vi "Data_select.vi"(8 "m":i32=2, 9 "P":i32=64, 10 "d(k) in":dbl[][](array[numeric]), 11 "g(k) in":dbl[][](array[numeric])) -> (1 "d(k) lineal":ext[](array[numeric]), 3 "g(k) lineal":ext[](array[numeric]))   [LabVIEW 2015]
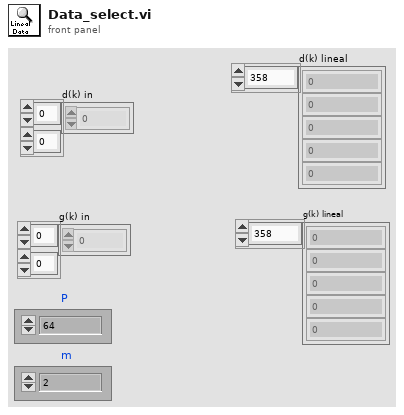
[diagram p1: front panel]
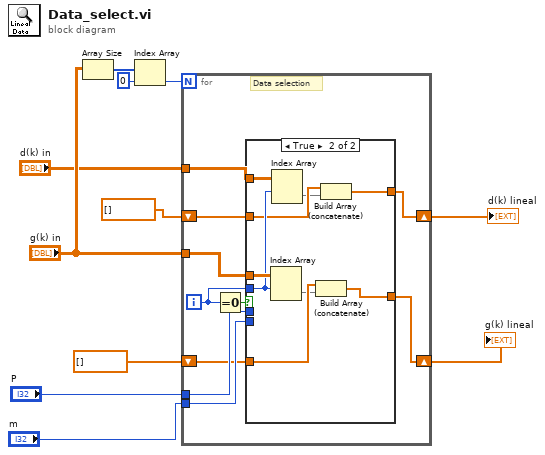
[diagram p0: block diagram]
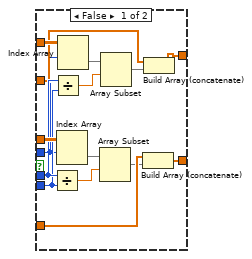
[diagram p2: hidden frame]
diagram:
  n1 = Array Size(array="g(k) in") -> (size(s)=w10:i32[])
  n2 = Index Array(array=w10, index=0) -> (element=w8:i32)
  n3 = for {
    N: w8 -> [_]
    tunnel: "g(k) in" -> [w20]
    tunnel: "m" -> [w18]
    tunnel: "P" -> [w17]
    shift-right: [w15] -> w4
    shift-left: ext[] [] ("Photon trace A") -> [w16]
    tunnel: "d(k) in" -> [w14]
    shift-right: [w12] -> w1
    shift-left: ext[] [] ("Photon trace A") -> [w13]
    i -> [w19]
    # "Data selection"
    n4 = Equal To 0?(x=w19) -> (x = 0?=w21:bool)
    n5 = case shown="True" w21 {
      tunnel: w20 -> [w36 w45]
      tunnel: w19 -> [w22 w40]
      tunnel: w18 -> [w25 _]
      tunnel: w17 -> [w26 _]
      tunnel: w16 -> [w34 w44]
      tunnel: [w35 w42] -> w15
      tunnel: w14 -> [w27 w41]
      tunnel: w13 -> [w23 w39]
      tunnel: [w24 w37] -> w12
      frame False {
        n6 = Divide(x=w26, y=w25) -> (x/y=w32:dbl)
        n7 = Divide(x=w26, y=w25) -> (x/y=w29:dbl)
        n8 = Index Array(array=w36, index (row)=w22) -> (element=w33:dbl[])  [unwired: 1 in]
        n9 = Index Array(array=w27, index (row)=w22) -> (element=w30:dbl[])  [unwired: 1 in]
        n10 = Array Subset(array=w33, index=w32) -> (w31:dbl[])  [unwired: 1 in]
        n11 = Array Subset(array=w30, index=w29) -> (w28:dbl[])  [unwired: 1 in]
        n12 = Build Array (concatenate)(w34, w31) -> (w35:ext[])
        n13 = Build Array (concatenate)(w23, w28) -> (w24:ext[])
      }
      frame True {
        n14 = Index Array(array=w45, index (row)=w40) -> (element=w43:dbl[])  [unwired: 1 in]
        n15 = Index Array(array=w41, index (row)=w40) -> (element=w38:dbl[])  [unwired: 1 in]
        n16 = Build Array (concatenate)(w44, w43) -> (w42:ext[])
        n17 = Build Array (concatenate)(w39, w38) -> (w37:ext[])
      }
    }
  }
  "g(k) lineal" <- w4
  "d(k) lineal" <- w1
